vi "scan current(SubVI).vi"(1 "Current":dbl=300.0, 6 "data":refnum<queue>, 7 "Current 2":dbl=300.0, 9 "steps number":i32, 15 "config":refnum<queue>) -> (8 "错误输出":errorcluster)   [LabVIEW 2019, in "SubVI.lvlib"]
uses:
  SubVI.lvlib
  config.ctl
  Instrument.ctl
  lib/QDInstrument.dll
  <vilib>/NI/Modbus Library/API/Master/Modbus Master.lvclass
panel:
  out "数组":dbl[](array[numeric])
  # "(真是通道1，假是通道2)"
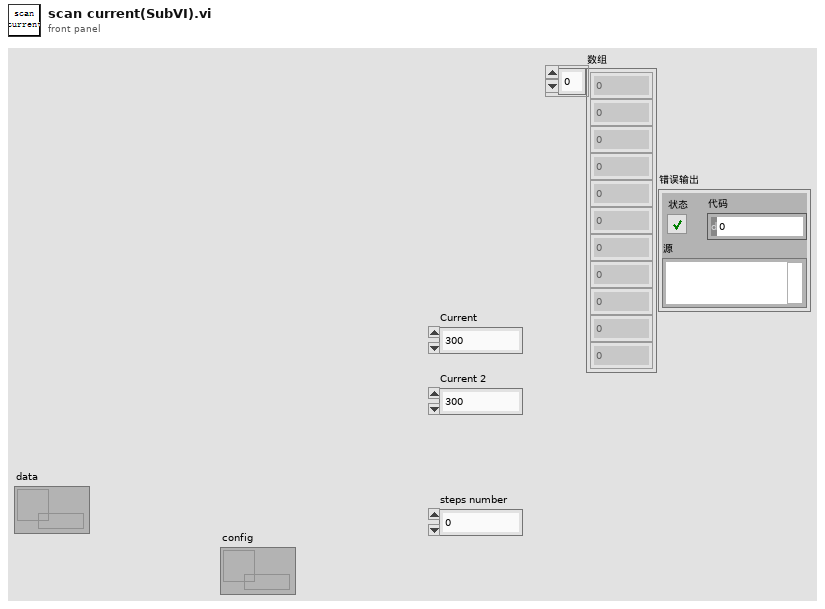
[diagram p1: front panel]
types:
  T1 = typedef "config.ctl" = cluster{"initialize":string, "6221":cluster{"6221 Resource":refnum<visa-resource-name>, "Delta status":bool}, "7001":cluster{"Ch":bool}, "SR830+6221":cluster{"source":u16, "阻抗":dbl, "量程入 4":i32, "量程入 3":i32, "量程入 2":i32, "量程入 1":i32, "电流":dbl, "SR830 2":bool, "SR830 3":bool, "SR830 4":bool, "SR830 1":bool, "VISA 1":refnum<visa-resource-name>, "VISA 2":refnum<visa-resource-name>, "VISA 3":refnum<visa-resource-name>, "VISA 4":refnum<visa-resource-name>, "量程":enum16{"量程每次测量会判定", "量程不变为设定值"}}, "2400":cluster{"2400":bool, "VISA":refnum<visa-resource-name>}, "ch":cluster{"ch str":string, "ch1":bool, "ch2":bool, "布尔":bool}, "error":bool, "数据文件路径":path, "log":cluster{"log路径":path, "log interval":dbl}, "Instrument":T2}
  T2 = typedef "Instrument.ctl" = cluster{"335 Resource":refnum<visa-resource-name>, "Input (0:A)":u16, "Instrument Type":i32, "quantum design":refnum<k24>, "Heater Output (1:1)":u16, "335state":refnum<vi>, "semaphore":T3, "TCP master instance":refnum<class "Modbus Master.lvclass">}
  T3 = typedef "Semaphore RefNum" = refnum<k1>
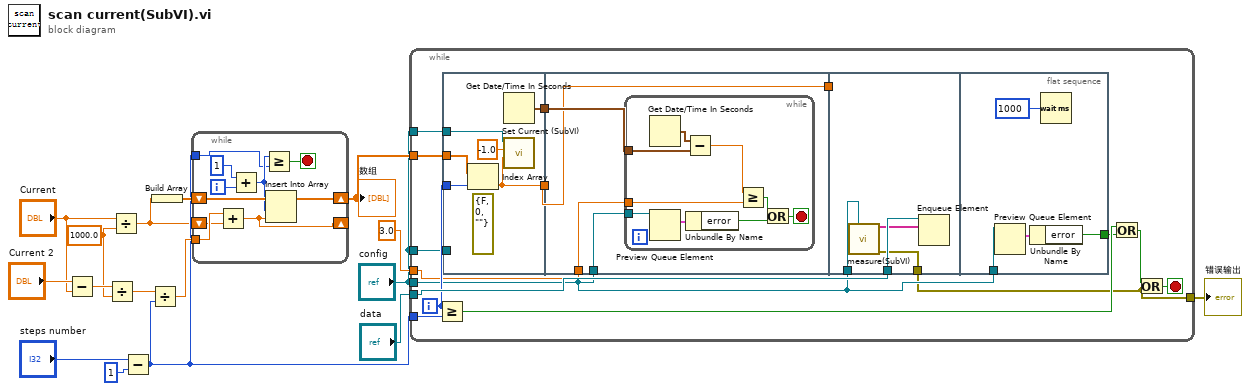
[diagram p0: block diagram]
diagram:
  w5 = 1000.0 ("y")
  n1 = Subtract(x="Current 2", y="Current") -> (x-y=w6:dbl)
  n2 = Divide(x=w6, y=w5) -> (x/y=w4:dbl)
  n3 = Divide(x="Current", y=w5) -> (x/y=w2:dbl)
  n4 = Subtract(x="steps number", y=1) -> (x-y=w9:i32)
  n5 = Divide(x=w4, y=w9) -> (x/y=w16:dbl)
  n6 = Build Array(w2) -> (w15:dbl[])
  n7 = while {
    shift-right: [w26] -> w13
    shift-left: w15 -> [w25]
    tunnel: w16 -> [w20]
    tunnel: w9 -> [w19]
    shift-right: [w18] -> _
    shift-left: w2 -> [w17]
    i -> [w24]
    stop <- w21 stop-if-true
    n8 = Add(x=w20, y=w17) -> (x+y=w18:dbl)
    n9 = Add(x=1, y=w24) -> (x+y=w22:i32)
    n10 = Greater Or Equal?(x=w22, y=w19) -> (x >= y?=w21:bool)
    n11 = Insert Into Array(array=w25, index=w22, new element=w18) -> (w26:dbl[])
  }
  "数组" <- w13
  n12 = while {
    tunnel: w9 -> [w40]
    tunnel: "data" -> [w42]
    tunnel: "config" -> [w33]
    tunnel: w13 -> [w38]
    tunnel: "config" -> [w37]
    tunnel: [w30] -> w12
    tunnel: 3.0 ("Delay") -> [w34]
    tunnel: "config" -> [w28]
    i -> [w39]
    stop <- w36 stop-if-true
    n13 = Greater Or Equal?(x=w39, y=w40) -> (x >= y?=w41:bool)
    n14 = flat-sequence {
      tunnel: w39 -> [w47]
      tunnel: w38 -> [w48]
      tunnel: w37 -> [_]
      tunnel: [w46] -> w35
      tunnel: [w44] -> w32
      tunnel: w28 -> [w45]
      tunnel: w35 -> [w52]
      tunnel: w34 -> [w51]
      tunnel: w33 -> [w50]
      tunnel: w32 -> [w49]
      tunnel: [w49] -> w31
      tunnel: w42 -> [w65]
      tunnel: [w64] -> w30
      tunnel: w33 -> [w63]
      tunnel: w31 -> [_]
      tunnel: w33 -> [w69]
      tunnel: [w66] -> w27
      frame #0 {
        (unwired) errorcluster {"status"=FALSE, "code"=0, "source"=""} ("error in (no error)")
        n15 = Index Array(array=w48, index=w47) -> (element=w44:dbl)
        n16 = Get Date/Time In Seconds() -> (seconds since 1Jan1904=w46:timestamp)
        n17 = call "Set Current (SubVI).vi"("current(A)"=w44, "freq"=-1.0, "队列输入"=w45) -> ()  [unwired: 9 in]
      }
      frame #1 {
        n18 = while {
          tunnel: w52 -> [w60]
          tunnel: w51 -> [w58]
          tunnel: w50 -> [w56]
          stop <- w55 stop-if-true
          n19 = Get Date/Time In Seconds() -> (seconds since 1Jan1904=w61:timestamp)
          n20 = Preview Queue Element(queue=w56) -> (element=w54:T1)  [unwired: 2 in, 3 out]
          n21 = Subtract(x=w61, y=w60) -> (x-y=w59:dbl)
          n22 = Unbundle By Name(w54) -> ("error"=w53:bool)
          n23 = Greater Or Equal?(x=w59, y=w58) -> (x >= y?=w57:bool)
          n24 = Or(x=w57, y=w53) -> (x .or. y?=w55:bool)
        }
      }
      frame #2 {
        n25 = call "measure(SubVI).vi"("config"=w63) -> ("data"=w62:string[], "error out"=w64:errorcluster)  [unwired: 13 in]
        n26 = Enqueue Element(queue=w65, element=w62) -> ()  [unwired: 2 in, 3 out]
      }
      frame #3 {
        n27 = Preview Queue Element(queue=w69) -> (element=w67:T1)  [unwired: 2 in, 3 out]
        n28 = Unbundle By Name(w67) -> ("error"=w66:bool)
        n29 = Wait (ms)(milliseconds to wait=u32 1000 ("等待时间（毫秒）")) -> ()  [unwired: 1 out]
      }
    }
    n30 = Or(x=w41, y=w27) -> (x .or. y?=w29:bool)
    n31 = Or(x=w29, y=w30) -> (x .or. y?=w36:bool)
  }
  "错误输出" <- w12
